vi "Basic 2.vi"() -> ()   [LabVIEW 2014, in "Arduino TFT.lvlib"]
uses:
  <vilib>/Aledyne-TSXperts/Arduino Compatible Compiler for LabVIEW/addons/Arduino TFT/Arduino TFT.lvlib
panel:
  out "Error Out":errorcluster
  in  "Error In":errorcluster
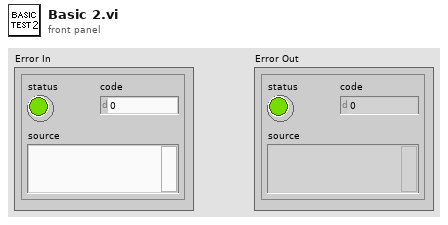
[diagram p1: front panel]
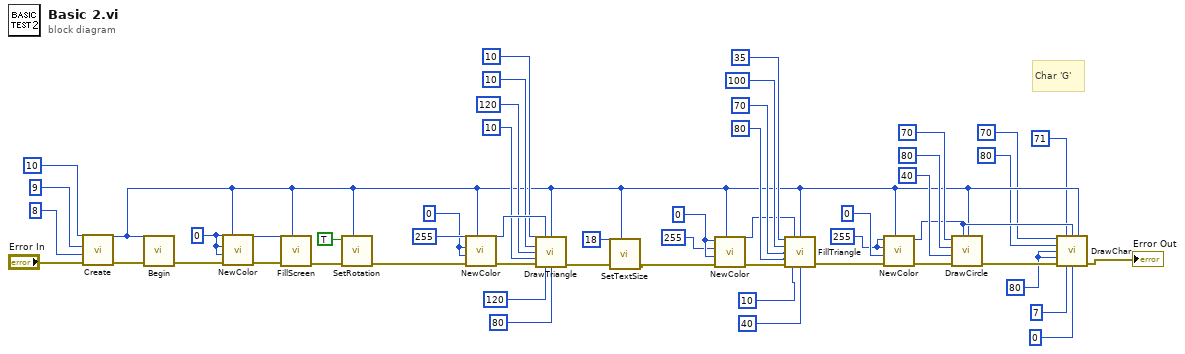
[diagram p0: block diagram]
diagram:
  w7 = i16 80 ("x")
  w2 = u8 255 ("red")
  w30 = u8 0 ("red")
  w34 = u8 0 ("red")
  w39 = u8 0 ("red")
  # "Char 'G'"
  n1 = call <vilib>:"Create.vi"("Error In"="Error In", "rst"=u8 8 ("cs"), "rs"=u8 9 ("cs"), "cs"=u8 10) -> ("Error Out"=w48:errorcluster, "Instance"=w11:u32)  [unwired: 4 in]
  n2 = call <vilib>:"Begin.vi"("Error In"=w48, "Instance"=w11) -> ("Error Out"=w38:errorcluster)  [unwired: 8 in]
  n3 = call <vilib>:"NewColor.vi"("Instance"=w11, "Error In"=w38, "blue"=w39, "green"=w39, "red"=w39) -> ("Error Out"=w37:errorcluster, "color"=w36:u16)  [unwired: 5 in]
  n4 = call <vilib>:"FillScreen.vi"("Instance"=w11, "Error In"=w37, "color"=w36) -> ("Error Out"=w20:errorcluster)  [unwired: 8 in]
  n5 = call <vilib>:"SetRotation.vi"("Instance"=w11, "Error In"=w20, "rotate 90deg?"=TRUE) -> ("Error Out"=w19:errorcluster)  [unwired: 8 in]
  n6 = call <vilib>:"NewColor.vi"("Instance"=w11, "Error In"=w19, "blue"=w34, "green"=w34, "red"=u8 255) -> ("Error Out"=w47:errorcluster, "color"=w46:u16)  [unwired: 5 in]
  n7 = call <vilib>:"DrawTriangle.vi"("x"=i16 10, "color"=w46, "Instance"=w11, "y"=i16 10 ("x"), "x2"=i16 120 ("x"), "y2"=i16 10 ("x"), "Error In"=w47, "x3"=i16 120 ("x"), "y3"=i16 80 ("x")) -> ("Error Out"=w33:errorcluster)  [unwired: 6 in]
  n8 = call <vilib>:"SetTextSize.vi"("Instance"=w11, "Error In"=w33, "size"=u8 18) -> ("Error Out"=w31:errorcluster)  [unwired: 8 in]
  n9 = call <vilib>:"NewColor.vi"("Instance"=w11, "Error In"=w31, "blue"=w30, "green"=u8 255 ("red"), "red"=w30) -> ("Error Out"=w24:errorcluster, "color"=w23:u16)  [unwired: 5 in]
  n10 = call <vilib>:"FillTriangle.vi"("x"=i16 35, "color"=w23, "Instance"=w11, "y"=i16 100 ("x"), "x2"=i16 70 ("x"), "y2"=i16 80 ("x"), "Error In"=w24, "x3"=i16 10 ("x"), "y3"=i16 40 ("x")) -> ("Error Out"=w14:errorcluster)  [unwired: 6 in]
  n11 = call <vilib>:"NewColor.vi"("Instance"=w11, "Error In"=w14, "blue"=u8 0 ("red"), "green"=w2, "red"=w2) -> ("Error Out"=w18:errorcluster, "color"=w12:u16)  [unwired: 5 in]
  n12 = call <vilib>:"DrawCircle.vi"("Instance"=w11, "color"=w12, "Error In"=w18, "r"=i16 40 ("x"), "y"=i16 80 ("x"), "x"=i16 70) -> ("Error Out"=w13:errorcluster)  [unwired: 5 in]
  n13 = call <vilib>:"DrawChar.vi"("x"=i16 70, "char"=u8 71, "char color"=w12, "Instance"=w11, "y"=i16 80 ("x"), "width"=w7, "height"=w7, "Error In"=w13, "pixel size"=u8 7 ("size"), "background color"=u16 0 ("bg")) -> ("Error Out"=→"Error Out":errorcluster)  [unwired: 5 in]
